vi "Get Oldest of ReaderTimestamps.vi"(11 "data attributes":variant) -> (1 "timestamp":timestamp format="%<%H:%M:%S%6u\n%x>T", 2 "reader ID":string, 3 "data attributes":variant)   [LabVIEW 2017]
uses:
  <vilib>/addons/_NISVFA/_Shared subVIs/Common/sv_Get NI Property Name String.vi
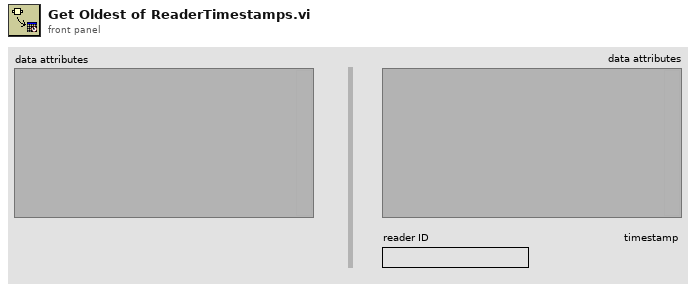
[diagram p1: front panel]
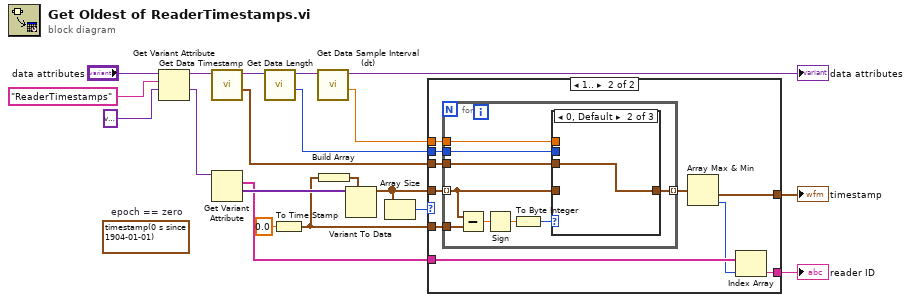
[diagram p0: block diagram]
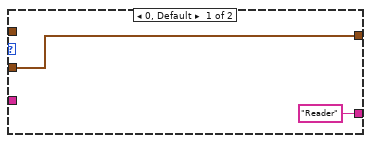
[diagram p2: hidden frame]
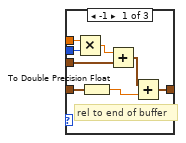
[diagram p3: hidden frame]
diagram:
  (unwired) timestamp(0 s since 1904-01-01)  # epoch == zero
  n1 = Get Variant Attribute(Variant="data attributes", name="ReaderTimestamps", default value (empty Variant)=variant ("ReaderTimestamps")) -> (duplicate Variant=w12:variant, value=w17:variant)  [unwired: 1 in, 2 out]
  n2 = call <vilib>:"Get Data Timestamp.vi"("variant in"=w12) -> ("timestamp"=w10:timestamp, "variant out"=w14:variant)  [unwired: 9 in]
  n3 = Get Variant Attribute(Variant=w17) -> (names=w6:string[], values=w16:variant[])  [unwired: 3 in, 2 out]
  n4 = call <vilib>:"Get Data Length.vi"("variant in"=w14) -> ("number of samples"=w9:i32, "variant out"=w13:variant)  [unwired: 9 in]
  n5 = To Time Stamp(1:0.0 ("number")) -> (0:w1:timestamp)
  n6 = call <vilib>:"Get Data Sample Interval (dt).vi"("variant in"=w13) -> ("dt [s]"=w8:dbl, "variant out"=→"data attributes":variant)  [unwired: 9 in]
  n7 = Build Array(w1) -> (w15:timestamp[])
  n8 = Variant To Data(type=w15, Variant=w16) -> (data=w4:timestamp[])  [unwired: 1 in, 1 out]
  n9 = Array Size(array=w4) -> (size(s)=w3:i32)
  n10 = case shown="1.." w3 {
    tunnel: w4 -> [_ w32]
    tunnel: w1 -> [w22 w31]
    tunnel: w10 -> [_ w30]
    tunnel: w9 -> [_ w29]
    tunnel: w8 -> [_ w28]
    tunnel: [w22 w26] -> w7
    tunnel: w6 -> [_ w25]
    tunnel: ["Reader" w23] -> w5
    frame 0, Default {
    }
    frame 1.. {
      n11 = for {
        tunnel: w32 -> [w36] mode=indexing
        tunnel: w31 -> [w41]
        tunnel: w30 -> [w37]
        tunnel: [w35] -> w27 mode=indexing
        tunnel: w29 -> [w34]
        tunnel: w28 -> [w33]
        n12 = Subtract(x=w36, y=w41) -> (x-y=w39:dbl)
        n13 = Sign(1:w39) -> (0:w40:dbl)
        n14 = To Byte Integer(number=w40) -> (8bit integer=w38:i8)
        n15 = case shown="0, Default" w38 {
          tunnel: w37 -> [w49 w50 _]
          tunnel: w36 -> [w44 _ w51]
          tunnel: [w42 w50 w51] -> w35
          tunnel: w34 -> [w47 _ _]
          tunnel: w33 -> [w46 _ _]
          frame -1 {
            # "rel to end of buffer"
            n16 = Multiply(x=w46, y=w47) -> (x*y=w48:dbl)
            n17 = To Double Precision Float(number=w44) -> (double precision float=w43:dbl)
            n18 = Add(x=w48, y=w49) -> (x+y=w45:timestamp)
            n19 = Add(x=w45, y=w43) -> (x+y=w42:timestamp)
          }
          frame 0, Default {
          }
          frame 1 {
          }
        }
      }
      n20 = Array Max & Min(array=w27) -> (min value=w26:timestamp, min index (indices)=w24:i32)  [unwired: 2 out]
      n21 = Index Array(array=w25, index=w24) -> (element=w23:string)
    }
  }
  "timestamp" <- w7
  "reader ID" <- w5
